vi "Register Notifier.vi"(8 "error in (no error)":errorcluster, 9 "ID In":variant, 10 "Notifier In":refnum<class "Notifier.lvclass">, 11 "Simple Map Notifier Controller in":refnum<class "Simple Map SEQ I64 Notifier Controller.lvclass">) -> (0 "error out":errorcluster, 3 "Simple Map Notifier Controller out":refnum<class "Simple Map SEQ I64 Notifier Controller.lvclass">)   [LabVIEW 2022 SP3, in "Simple Map SEQ I64 Notifier Controller.lvclass"]
uses:
  Simple Map SEQ I64 Notifier Controller.lvclass
  Ancestor Class/Actor Assistant/Notifier/Notifier.lvclass
  Simple Map SEQ I64 Notifier Controller.lvclass/Simple Map SEQ I64 Notifier Controller.ctl
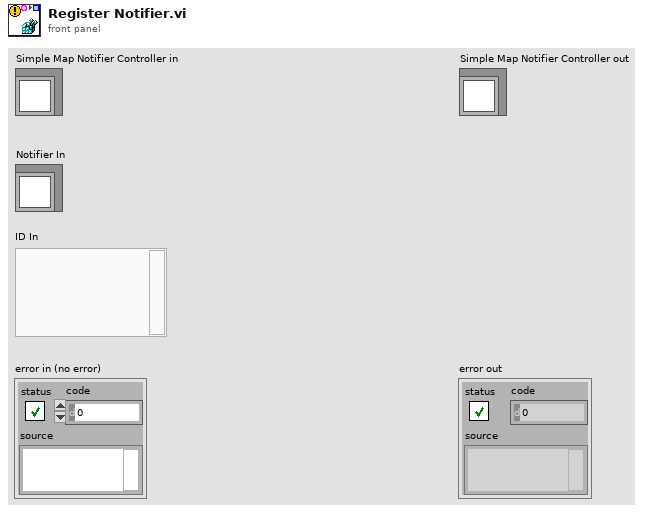
[diagram p1: front panel]
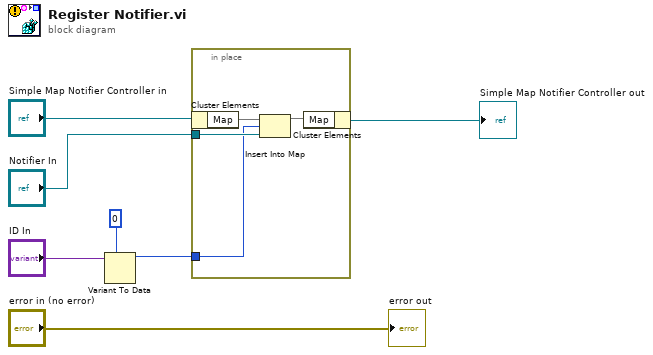
[diagram p0: block diagram]
diagram:
  n1 = Variant To Data(type=i64 0, Variant="ID In") -> (data=w1:i64)  [unwired: 1 in, 1 out]
  n2 = in-place {
    in-place-border: "Notifier In" -> [w9]
    in-place-border: w1 -> [w8]
    n3 = in-place-cluster #1("Simple Map Notifier Controller in") -> ("Map"=w11:map{i64, refnum<class "Notifier.lvclass">})
    n4 = Insert Into Map(map in=w11, key=w8, value=w9) -> (map out=w10:map{i64, refnum<class "Notifier.lvclass">})  [unwired: 2 out]
    n5 = in-place-cluster #1("Map"=w10) -> (→"Simple Map Notifier Controller out":refnum<class "Simple Map SEQ I64 Notifier Controller.lvclass">)
  }
  "error out" <- "error in (no error)"
